vi "Core.vi"(4 "CD_sensitivity %":i8(slide)=90 min=0 max=100 scale=0.1..100.0, 6 "Clouds":bool, 7 "Auto Balance":bool, 8 "Real-time Values":dbl[](array[numeric]), 9 "Loops":u8=3 min=1, 10 "Pointer Tolerance":i8(slide)=1 min=1 max=100 step=1 scale=1.0..11.0, 11 "Data in":T1={"[V]"=0.0, "Vertical sum"=0.0, "Horizontal sum"=0.0, "auto Loopback"=FALSE, "Auto Balance"=FALSE, "Out Cmd"=0, "Motor Cmd"=0, "ADC Values"=[], "Clouds ctrl"=FALSE, "Cloud Det"=FALSE, "Cloud Sens"=0, "Loops"=0, "VISA res"="COM3"}) -> (0 "Clouds detected":bool, 1 "Horizontal sum":dbl, 2 "Vertical sum":dbl, 3 "Data out":T1={"[V]"=0.0, "Vertical sum"=0.0, "Horizontal sum"=0.0, "auto Loopback"=FALSE, "Auto Balance"=FALSE, "Out Cmd"=0, "Motor Cmd"=0, "ADC Values"=[], "Clouds ctrl"=FALSE, "Cloud Det"=FALSE, "Cloud Sens"=0, "Loops"=0, "VISA res"="COM3"}, 5 "[V]":dbl=0.0023)   [LabVIEW 2014]
uses:
  Ctrls/Data cluster.ctl
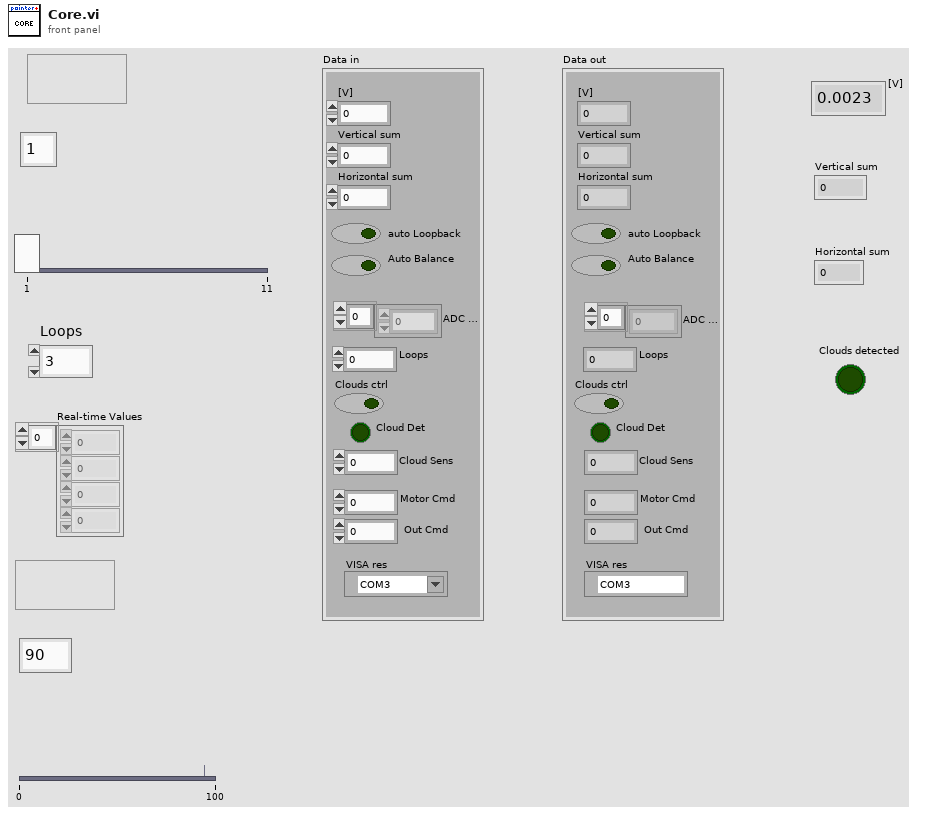
[diagram p1: front panel]
types:
  T1 = typedef "Data cluster.ctl" = cluster{"[V]":dbl, "Vertical sum":dbl, "Horizontal sum":dbl, "auto Loopback":bool, "Auto Balance":bool, "Out Cmd":i32, "Motor Cmd":i32, "ADC Values":dbl[], "Clouds ctrl":bool, "Cloud Det":bool, "Cloud Sens":i8, "Loops":u8, "VISA res":refnum<visa-resource-name>}
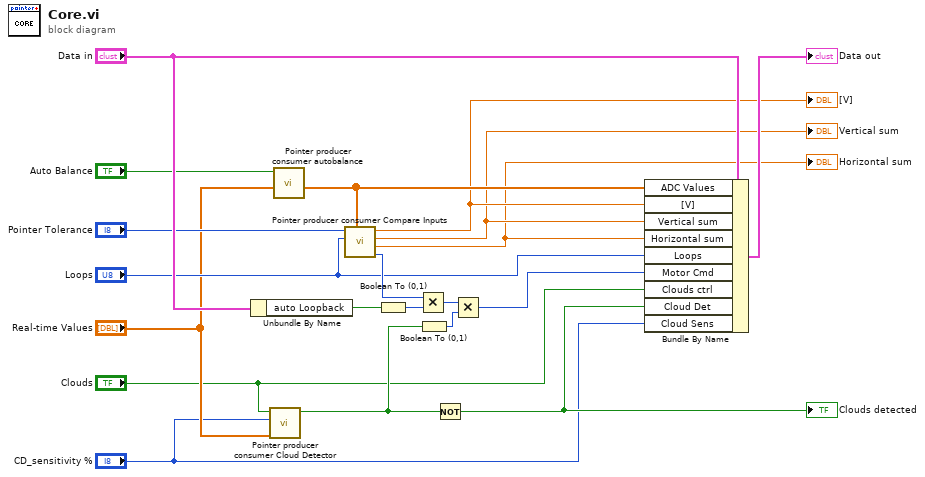
[diagram p0: block diagram]
diagram:
  n1 = Unbundle By Name("Data in") -> ("auto Loopback"=w10:bool)
  n2 = call "Pointer producer consumer Cloud Detector.vi"("Real-time Values"="Real-time Values", "Cloud Sensitivity"="CD_sensitivity %", "Cloud Ctrl"="Clouds") -> ("Cloud Detector"=w7:bool)  [unwired: 8 in]
  n3 = call "Pointer producer consumer autobalance.vi"("Real-time Values"="Real-time Values", "Auto Balance"="Auto Balance") -> ("New ADC Values"=w16:dbl[])  [unwired: 8 in, 1 out]
  n4 = call "Pointer producer consumer Compare Inputs.vi"("ADC in"=w16, "Loops"="Loops", "Tolerance IN"="Pointer Tolerance") -> ("motor"=w12:i32, "Horizontal summary"=w1:dbl, "Vertical summary"=w2:dbl, "Tolerance (V)"=w3:dbl)  [unwired: 5 in]
  "[V]" <- w3
  "Vertical sum" <- w2
  "Horizontal sum" <- w1
  n5 = Boolean To (0,1)(Boolean=w10) -> (0, 1=w15:i16)
  n6 = Multiply(x=w12, y=w15) -> (x*y=w13:i32)
  n7 = Boolean To (0,1)(Boolean=w7) -> (0, 1=w14:i16)
  n8 = Not(x=w7) -> (.not. x?=w5:bool)
  "Clouds detected" <- w5
  n9 = Multiply(x=w13, y=w14) -> (x*y=w8:i32)
  n10 = Bundle By Name(cluster="Data in", "ADC Values"=w16, "[V]"=w3, "Vertical sum"=w2, "Horizontal sum"=w1, "Loops"="Loops", "Motor Cmd"=w8, "Clouds ctrl"="Clouds", "Cloud Det"=w5, "Cloud Sens"="CD_sensitivity %") -> (→"Data out":T1)
